vi "RBL MAIN offline.vi"() -> ()   [LabVIEW 2015]
panel:
  out "even inner outer":bool
  out "even inner":bool
  out "BRAKE OIL SPIL":bool
  out "RESERVOIR LEAK":bool
  out "UNEVEN INNER":bool
  out "UNEVEN IO":bool
  out "GOOD":bool
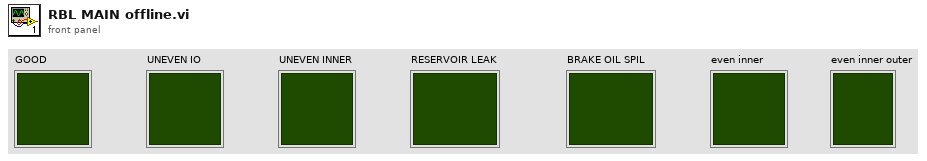
[diagram p1: front panel]
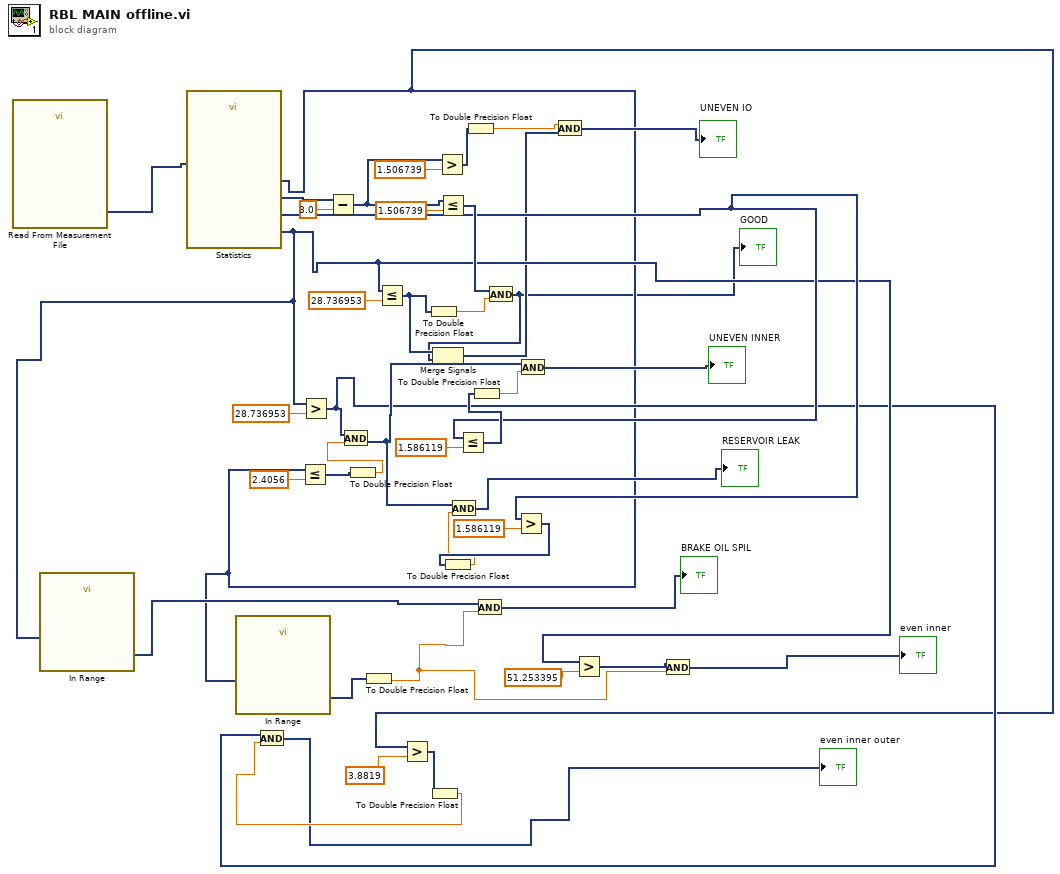
[diagram p0: block diagram]
diagram:
  n1 = call "Read From Measurement File"() -> ("Signals"=w8:dynamicdata)  [unwired: 6 in, 5 out]
  n2 = call "Statistics"("Signals"=w8) -> ("Skewness"=w21:dynamicdata, "Kurtosis"=w42:dynamicdata, "Standard Dev"=w6:dynamicdata, "Range"=w14:dynamicdata)  [unwired: 22 in, 1 out]
  n3 = call "In Range"("Operand 1"=w14) -> ("Result"=w16:dynamicdata)  [unwired: 9 in, 1 out]
  n4 = call "In Range"("Operand 1"=w6) -> ("Result"=w17:dynamicdata)  [unwired: 9 in, 1 out]
  n5 = Less Or Equal?(x=w6, y=2.4056) -> (x <= y?=w29:dynamicdata)
  n6 = Greater?(x=w14, y=28.736953) -> (0:w7:dynamicdata)
  n7 = Subtract(x=w42, y=3.0) -> (x-y=w37:dynamicdata)
  n8 = To Double Precision Float(number=w29) -> (double precision float=w28:dbl)
  n9 = And(x=w7, y=w28) -> (x .and. y?=w22:dynamicdata)
  n10 = To Double Precision Float(number=w17) -> (double precision float=w11:dbl)
  n11 = Less Or Equal?(x=w14, y=28.736953) -> (x <= y?=w33:dynamicdata)
  n12 = Greater?(x=w6, y=3.8819) -> (0:w5:dynamicdata)
  n13 = To Double Precision Float(number=w33) -> (double precision float=w40:dbl)
  n14 = To Double Precision Float(number=w5) -> (double precision float=w4:dbl)
  n15 = And(x=w7, y=w4) -> (x .and. y?=→"even inner outer":dynamicdata)
  n16 = Greater?(x=w37, y=1.506739) -> (0:w35:dynamicdata)
  n17 = Less Or Equal?(x=w37, y=1.506739) -> (x <= y?=w38:dynamicdata)
  n18 = Less Or Equal?(x=w21, y=1.586119) -> (x <= y?=w26:dynamicdata)
  n19 = To Double Precision Float(number=w35) -> (double precision float=w34:dbl)
  n20 = To Double Precision Float(number=w26) -> (double precision float=w25:dbl)
  n21 = And(x=w16, y=w11) -> (x .and. y?=→"BRAKE OIL SPIL":dynamicdata)
  n22 = And(x=w38, y=w40) -> (x .and. y?=w1:dynamicdata)
  "GOOD" <- w1
  n23 = Merge Signals(w33, w1) -> (w2:dynamicdata)
  n24 = Greater?(x=w21, y=1.586119) -> (0:w20:dynamicdata)
  n25 = To Double Precision Float(number=w20) -> (double precision float=w19:dbl)
  n26 = And(x=w22, y=w19) -> (x .and. y?=→"RESERVOIR LEAK":dynamicdata)
  n27 = And(x=w22, y=w25) -> (x .and. y?=→"UNEVEN INNER":dynamicdata)
  n28 = And(x=w34, y=w2) -> (x .and. y?=→"UNEVEN IO":dynamicdata)
  n29 = Greater?(x=w14, y=51.253395) -> (0:w12:dynamicdata)
  n30 = And(x=w12, y=w11) -> (x .and. y?=→"even inner":dynamicdata)
